vi "刀具点.vi"(6 "error in (no error)":errorcluster caption="错误输入（无错误）", 9 "Scene Object In":refnum<vi> caption="场景对象输入") -> (0 "error out":errorcluster caption="错误输出", 3 "Scene Object Out":refnum<vi> caption="场景对象输出")   [LabVIEW 2019]
uses:
  <vilib>/picture/3D Picture Control/Object/Create Object (drawable).vi
  <vilib>/picture/3D Picture Control/Object/Add Object (no reference).vi
  <vilib>/picture/3D Picture Control/NI_3D Picture Control.lvlib
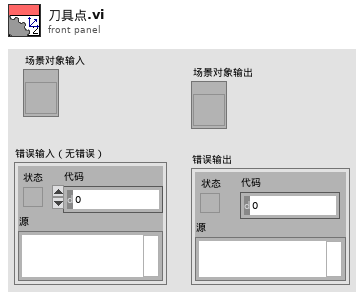
[diagram p1: front panel]
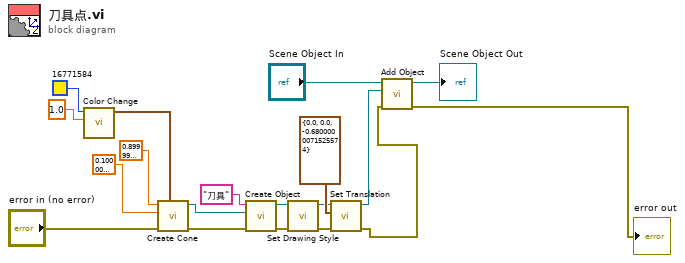
[diagram p0: block diagram]
diagram:
  n1 = call <vilib>:"Color Change.vi"("Alpha"=1.0, "Color"=u32 16771584) -> ("RGBA"=w14:cluster{"R":sgl, "G":sgl, "B":sgl, "A":sgl})  [unwired: 9 in]
  n2 = call <vilib>:"Create Cone.vi"("Color"=w14, "error in (no error)"="error in (no error)", "Radius"=sgl 0.1, "Height"=sgl 0.9) -> ("error out"=w13:errorcluster, "New Cone Refnum"=w18:refnum<vi>)  [unwired: 6 in]
  n3 = call-poly <vilib>:"Create Object.vi"("error in (no error)"=w13, "Geometry"=w18, "Name"="刀具") -> ("error out"=w12:errorcluster, "Scene:New Object"=w17:refnum<vi>)  [unwired: 7 in]
  n4 = call <vilib>:"Set Drawing Style.vi"("error in (no error)"=w12, "Scene Object In"=w17) -> ("error out"=w9:errorcluster, "Scene Object Out"=w10:refnum<vi>)  [unwired: 8 in]
  n5 = call <vilib>:"Set Translation.vi"("error in (no error)"=w9, "Translation"=cluster{"X":sgl, "Y":sgl, "Z":sgl} {"X"=0.0, "Y"=0.0, "Z"=-0.68}, "Scene Object"=w10) -> ("error out"=w2:errorcluster, "Translated Object"=w6:refnum<vi>)  [unwired: 7 in]
  n6 = call-poly <vilib>:"Add Object.vi"("error in (no error)"=w2, "New Object In"=w6, "Scene Object In"="Scene Object In") -> ("error out"=→"error out":errorcluster, "Scene Object Out"=→"Scene Object Out":refnum<vi>)  [unwired: 7 in]
